vi "4.7.vi"() -> ()   [LabVIEW 2017]
panel:
  out "猜测次数值":dbl
  out "随机的数":dbl
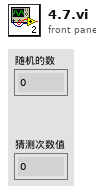
[diagram p1: front panel]
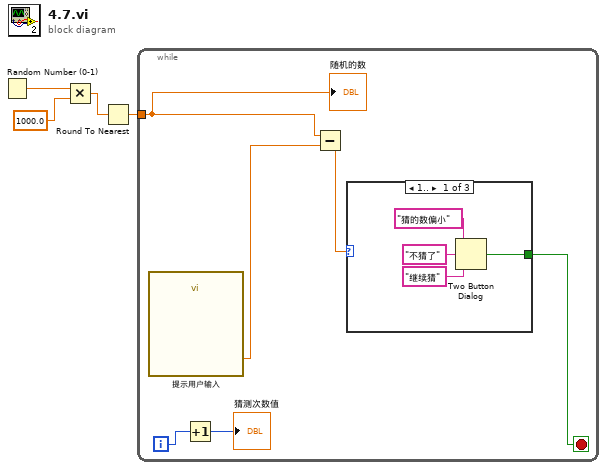
[diagram p0: block diagram]
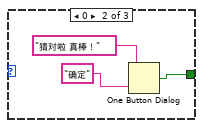
[diagram p2: hidden frame]
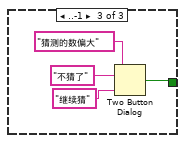
[diagram p3: hidden frame]
diagram:
  n1 = Random Number (0-1)() -> (number: 0 to 1=w3:dbl)
  n2 = Multiply(x=w3, y=1000.0) -> (x*y=w4:dbl)
  n3 = Round To Nearest(number=w4) -> (nearest integer value=w1:dbl)
  n4 = while {
    tunnel: w1 -> [w5]
    i -> [w7]
    stop <- w10 stop-if-true
    n5 = call "提示用户输入"() -> ("请在1-1000猜"=w8:dbl)  [unwired: 17 in, 2 out]
    n6 = Increment(x=w7) -> (x+1=→"猜测次数值":i32)
    n7 = Subtract(x=w5, y=w8) -> (x-y=w9:dbl)
    n8 = case shown="1.." w9 {
      tunnel: [w11 w15 w19] -> w10
      frame 1.. {
        n9 = Two Button Dialog(message="猜的数偏小" ("消息"), 1:"继续猜" ("F按钮名称（“取消”）"), 2:"不猜了" ("T按钮名称（“确定”）")) -> (T button?=w11:bool)
      }
      frame 0 {
        n10 = One Button Dialog(message="猜对啦 真棒！" ("消息"), button name ("OK")="确定" ("T按钮名称（“确定”）")) -> (true=w15:bool)
      }
      frame ..-1 {
        n11 = Two Button Dialog(message="猜测的数偏大" ("消息"), 1:"继续猜" ("F按钮名称（“取消”）"), 2:"不猜了" ("T按钮名称（“确定”）")) -> (T button?=w19:bool)
      }
    }
    "随机的数" <- w5
  }
